vi "set FPGA Resource Info.vi"(8 "error in (no error)":errorcluster, 10 "Value":variant, 11 "Relative Item Ref Out":T1 format="%.0x") -> (0 "error out":errorcluster, 3 "Item Ref out":T1 format="%.0x")   [LabVIEW 2016, in "FPGA Addon System Explorer.lvlib"]
uses:
  FPGA Addon System Explorer.lvlib
  <vilib>/NI Veristand/Custom Device API/Custom Device Item Ref.ctl
  <vilib>/NI Veristand/Custom Device API/Set Item Property (Variant).vi
  FPGA-Resource-Manager-APIs/Source/FPGA RM Client API.lvlib
  <vilib>/NI VeriStand/Custom Device API/Custom Device API.lvlib
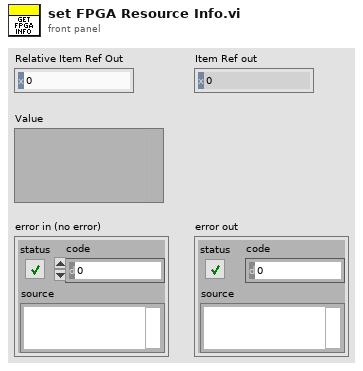
[diagram p1: front panel]
types:
  T1 = typedef "Custom Device API.lvlib/Custom Device Item Ref.ctl" = u64
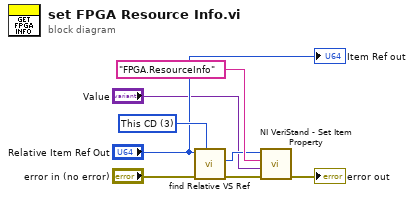
[diagram p0: block diagram]
diagram:
  w6 = u16 3 items=["Targets", "Controller", "Custom Devices", "This CD", "This CD/Group", "This CD/Group/SubGroup"] ("Relative Type")
  n1 = call "find Relative VS Ref.vi"("Relative Type"=w6, "error in (no error)"="error in (no error)", "Item Ref in"="Relative Item Ref Out") -> ("error out"=w2:errorcluster, "Relative Item Ref Out"=w3:T1)  [unwired: 4 in, 3 out]
  n2 = call-poly <vilib>:"NI VeriStand - Set Item Property.vi"("error in (no error)"=w2, "Value"="Value", "Property Name"="FPGA.ResourceInfo", "Item Ref in"=w3) -> ("error out"=→"error out":errorcluster)  [unwired: 5 in, 2 out]
  "Item Ref out" <- "Relative Item Ref Out"
